vi "TrajectoryConfig_GetStartVelocity.vi"(11 "inTRAJECTORY_CONFIG":T1 {"End Velocity" format="%20.4f"; "StartVelocity" format="%20.4f"; "Max Acceleration" format="%20.4f"; "MaxVelocity" format="%20.4f"}) -> (3 "StartVelocity":dbl)   [LabVIEW 2019, in "Trajectory_Library.lvlib"]
doc: "Updates the reversed flag in the Trajectory Config data structure.\n\nParameters:\n - InTrajectoryConfig - The trajectory configuration data structure\n - Reversed - Whether the trajectory should be reversed or not.\n\nReturns:\n - OutTrajectoryConfig - Modified trajectory configuration data structure"
uses:
  TypeDef/TRAJ_CONFIG.ctl
  Trajectory_Library.lvlib
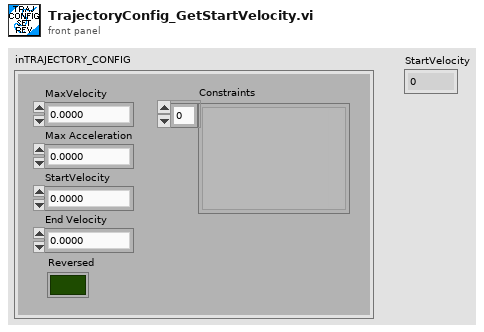
[diagram p1: front panel]
types:
  T1 = typedef "Trajectory_Library.lvlib/TRAJ_CONFIG.ctl" = cluster{"MaxVelocity":dbl, "Max Acceleration":dbl, "StartVelocity":dbl, "End Velocity":dbl, "Reversed":bool, "Constraints":variant[]}
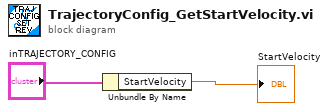
[diagram p0: block diagram]
diagram:
  n1 = Unbundle By Name("inTRAJECTORY_CONFIG") -> ("StartVelocity"=→"StartVelocity":dbl)
